vi "Prepare DAQmx Module.vi"(4 "Create Scaling (F)":bool, 6 "On Demand (F)":bool, 8 "error in (no error)":errorcluster, 10 "Group Config (Lookup)":refnum<class "Group Config.lvclass">, 11 "Module in":refnum<class "Module.lvclass">) -> (0 "error out":errorcluster, 1 "Scaling":refnum<class "Scaling.lvclass">, 2 "Group":refnum<class "Group DBL.lvclass">, 3 "Module out":refnum<class "Module.lvclass">, 5 "DAQmx Task":refnum<k21>, 7 "Sampling Config":T1)   [LabVIEW 2023, in "VolatusDAQ.lvlib"]
uses:
  VolatusDAQ.lvlib
  Volatus/Module/Module.lvclass
  lv-vecto/Vecto/Group DBL/Group DBL.lvclass
  VolatusDAQConfig/Sampling Config.ctl
  VolatusData/Scaling/Scaling.lvclass
  Volatus/Event Level.ctl
  Volatus/Module/Module.lvclass/Module.ctl
  VolatusConfig/VolatusConfigElement/VolatusConfigElement.lvclass/VolatusConfigElement.ctl
  Volatus/Module/Config.vi
  VolatusConfig/VolatusConfigElement/Element.vi
  VolatusConfig/Group/Group Config.lvclass
  VolatusConfig/Scaling/Create (Group).vi
  VolatusData/Scaling/Create (Config).vi
  <vilib>/DAQmx/configure/timing.llb/DAQmx Timing (Sample Clock).vi
  VolatusDAQConfig/DAQmxChannel/DAQmxChannel.lvclass
  VolatusConfig/Task/Task Config.lvclass
  VolatusDAQConfig/VolatusDAQConfig.lvlib
  Volatus/Volatus.lvlib
  VolatusConfig/VolatusConfigElement/VolatusConfigElement.lvclass
  VolatusConfig/Channel/Channel Config.lvclass
  C:/dev/volatus/mts-volatus-super/libs/lv-volatus/VolatusConfig/VolatusConfigElement/VolatusConfigElement.lvclass
  C:/dev/volatus/mts-volatus-super/libs/lv-volatus/VolatusConfig/Channel/Channel Config.lvclass
  C:/dev/volatus/mts-volatus-super/libs/lv-vecto/Vecto/Group/Group.lvclass
  C:/dev/volatus/mts-volatus-super/libs/lv-vecto/Vecto/Group DBL/Group DBL.lvclass
  C:/dev/volatus/mts-volatus-super/libs/lv-volatus/VolatusConfig/Group/Group Config.lvclass
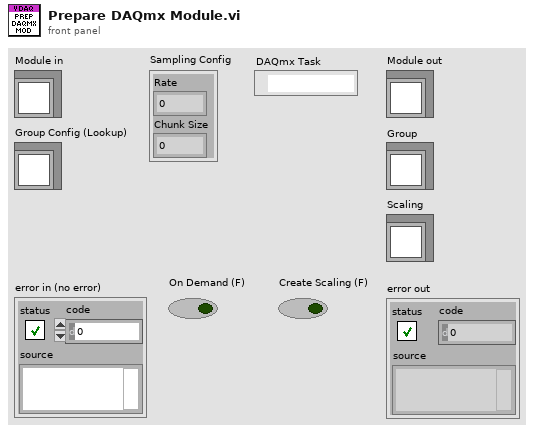
[diagram p1: front panel]
types:
  T1 = typedef "VolatusDAQConfig.lvlib/Sampling Config.ctl" = cluster{"Rate":dbl, "Chunk Size":i32}
  T2 = typedef "Volatus.lvlib/Event Level.ctl" = enum16{"Debug", "Info", "Warning", "Error"}
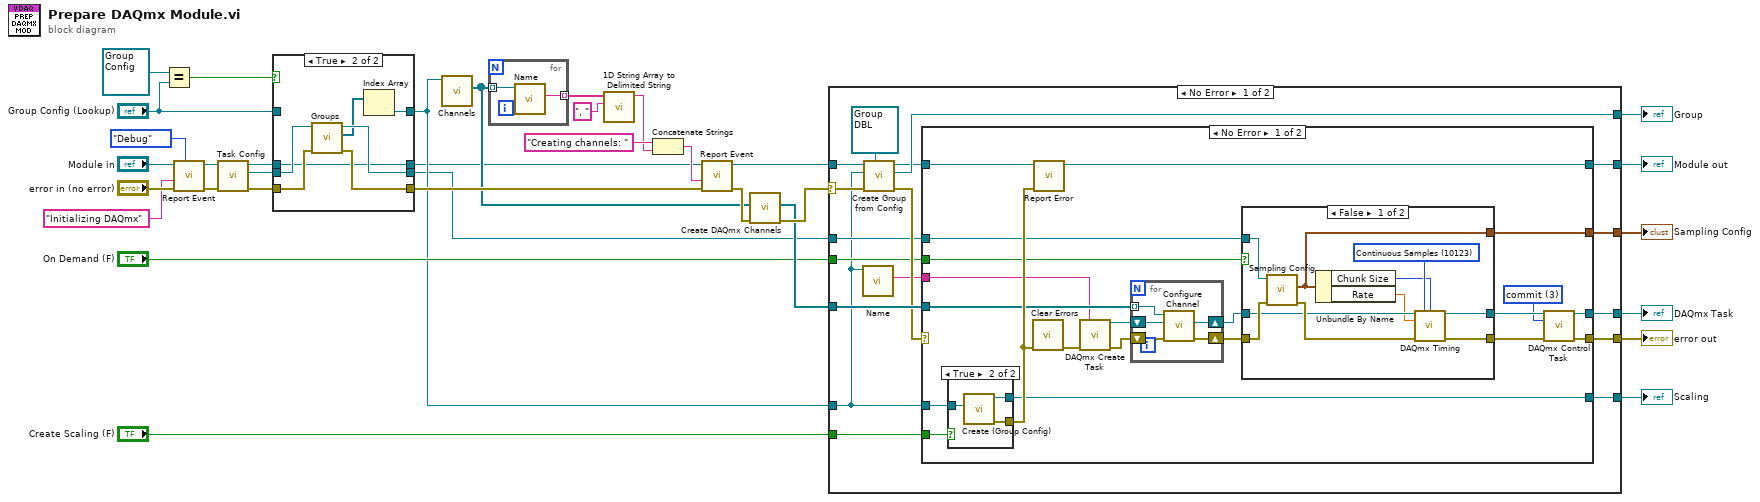
[diagram p0: block diagram]
diagram:
  n1 = Equal?(x=refnum<class "Group Config.lvclass"> refnum, y="Group Config (Lookup)") -> (x = y?=w6:bool)
  n2 = call "Report Event.vi"("Level (Info)"=Event_Level."Debug", "error in (no error)"="error in (no error)", "Message"="Initializing DAQmx", "Module in"="Module in") -> ("error out"=w18:errorcluster, "Module out"=w16:refnum<class "Module.lvclass">)  [unwired: 6 in]
  n3 = call "Task Config.vi"("error in (no error)"=w18, "Module in"=w16) -> ("error out"=w31:errorcluster, "Task Config"=w30:refnum<class "Task Config.lvclass">, "Module out"=w5:refnum<class "Module.lvclass">)  [unwired: 7 in]
  n4 = case shown="True" w6 {
    tunnel: [w36 w45] -> w34
    tunnel: w31 -> [w36 w44]
    tunnel: w30 -> [w35 w43]
    tunnel: [w35 w42] -> w3
    tunnel: [w38 w40] -> w19
    tunnel: "Group Config (Lookup)" -> [w38 _]
    tunnel: w5 -> [w37 w39]
    tunnel: [w37 w39] -> w2
    frame False {
    }
    frame True {
      n5 = call "Groups.vi"("error in (no error)"=w44, "Task in"=w43) -> ("error out"=w45:errorcluster, "Groups"=w41:refnum<class "Group Config.lvclass">[], "Task out"=w42:refnum<class "Task Config.lvclass">)  [unwired: 7 in]
      n6 = Index Array(array=w41) -> (element=w40:refnum<class "Group Config.lvclass">)  [unwired: 1 in]
    }
  }
  n7 = call "Channels.vi"("Group in"=w19) -> ("Channels"=w4:refnum<class "Channel Config.lvclass">[])  [unwired: 8 in, 2 out]
  n8 = for {
    tunnel: w4 -> [w47] mode=indexing
    tunnel: [w46] -> w13 mode=indexing
    n9 = call "Name.vi"("VolatusConfigElement in"=w47) -> ("Name"=w46:string)  [unwired: 8 in, 2 out]
  }
  n10 = call <vilib>:"1D String Array to Delimited String.vi"("delimiter"=", ", "string array"=w13) -> ("delimited string"=w9:string)  [unwired: 9 in]
  n11 = Concatenate Strings("Creating channels: " ("Message"), w9) -> (w8:string)
  n12 = call "Report Event.vi"("error in (no error)"=w34, "Message"=w8, "Module in"=w2) -> ("error out"=w33:errorcluster, "Module out"=w11:refnum<class "Module.lvclass">)  [unwired: 7 in]
  n13 = call "Create DAQmx Channels.vi"("error in (no error)"=w33, "Channels"=w4) -> ("error out"=w32:errorcluster, "DAQmxChannels"=w27:refnum<class "DAQmxChannel.lvclass">[])  [unwired: 8 in]
  n14 = case shown="No Error" w32 {
    selector: w32 -> [w64 w108]
    tunnel: w11 -> [w63 w109]
    tunnel: [w61 _] -> w28
    tunnel: w27 -> [w60 _]
    tunnel: [w59 _] -> w26
    tunnel: [w48 w109] -> w25
    tunnel: [w58 w108] -> w24
    tunnel: [w57 _] -> w23
    tunnel: "Create Scaling (F)" -> [w56 _]
    tunnel: "On Demand (F)" -> [w54 _]
    tunnel: [w53 _] -> w20
    tunnel: w3 -> [w52 _]
    tunnel: w19 -> [w51 _]
    frame No Error {
      n15 = call "Name.vi"("VolatusConfigElement in"=w51) -> ("Name"=w50:string)  [unwired: 8 in, 2 out]
      n16 = call "Create Group from Config.vi"("Group Type (Abstract)"=refnum<class "Group DBL.lvclass"> refnum ("Vecto.lvlib:Group.lvclass"), "error in (no error)"=w64, "Group Config"=w51, "Module in"=w63) -> ("error out"=w55:errorcluster, "Group"=w61:refnum<class "Group DBL.lvclass">, "Module out"=w49:refnum<class "Module.lvclass">)  [unwired: 5 in]
      n17 = case shown="No Error" w55 {
        selector: w55 -> [_ w107]
        tunnel: w60 -> [w79 _]
        tunnel: [w78 _] -> w59
        tunnel: [w77 w107] -> w58
        tunnel: w51 -> [w76 _]
        tunnel: [w75 _] -> w57
        tunnel: w56 -> [w74 _]
        tunnel: w54 -> [w73 _]
        tunnel: [w72 _] -> w53
        tunnel: w52 -> [w71 _]
        tunnel: w50 -> [w69 _]
        tunnel: w49 -> [w67 w106]
        tunnel: [w65 w106] -> w48
        frame No Error {
          w80 = 3 items=["verify"=2, "reserve"=4, "commit"=3, "unreserve"=5, "abort"=6] ("action")
          n18 = case shown="True" w74 {
            tunnel: w76 -> [_ w88]
            tunnel: [_ w87] -> w75
            tunnel: [_ w86] -> w85
            frame False {
            }
            frame True {
              n19 = call "Create (Group Config).vi"("Group Config"=w88) -> ("error out"=w86:errorcluster, "Scaling out"=w87:refnum<class "Scaling.lvclass">)  [unwired: 9 in]
            }
          }
          n20 = call <vilib>:"Clear Errors.vi"("error in (no error)"=w85) -> ("error out"=w66:errorcluster)  [unwired: 5 in, 1 out]
          n21 = call "Report Error.vi"("error in (no error)"=w85, "Module in"=w67) -> ("Module out"=w65:refnum<class "Module.lvclass">)  [unwired: 8 in, 1 out]
          n22 = call <vilib>:"DAQmx Create Task.vi"("new task name"=w69, "error in"=w66) -> ("task out"=w70:refnum<k21>, "error out"=w68:errorcluster)  [unwired: 12 in]
          n23 = for {
            shift-right: [w91] -> w83
            shift-left: w70 -> [w92]
            tunnel: w79 -> [w93] mode=indexing
            shift-right: [w89] -> w84
            shift-left: w68 -> [w90]
            n24 = call-dynamic "Configure Channel.vi"("error in (no error)"=w90, "DAQmx Task In"=w92, "DAQmxChannel in"=w93) -> ("error out"=w89:errorcluster, "DAQmx Task"=w91:refnum<k21>)  [unwired: 7 in]
          }
          n25 = case shown="False" w73 {
            tunnel: w84 -> [w102 w104]
            tunnel: w83 -> [w101 w105]
            tunnel: [w99 w104] -> w82
            tunnel: [w98 w105] -> w81
            tunnel: [w95 _] -> w72
            tunnel: w71 -> [w94 _]
            frame False {
              w100 = 10123 items=["Finite Samples"=10178, "Continuous Samples"=10123, "Hardware Timed Single Point"=12522] ("sample mode")
              n26 = call "Sampling Config.vi"("error in (no error)"=w102, "Task In"=w94) -> ("error out"=w103:errorcluster, "Sampling Config"=w95:T1)  [unwired: 7 in, 1 out]
              n27 = Unbundle By Name(w95) -> ("Chunk Size"=w96:i32, "Rate"=w97:dbl)
              n28 = call-poly <vilib>:"DAQmx Timing.vi"("task/channels in"=w101, "sample mode"=w100, "samples per channel"=w96, "rate"=w97, "error in"=w103) -> ("task out"=w98:refnum<k21>, "error out"=w99:errorcluster)  [unwired: 9 in]
            }
            frame True {
            }
          }
          n29 = call <vilib>:"DAQmx Control Task.vi"("task/channels in"=w81, "action"=w80, "error in"=w82) -> ("task out"=w78:refnum<k21>, "error out"=w77:errorcluster)  [unwired: 11 in]
        }
        frame Error {
        }
      }
    }
    frame Error {
    }
  }
  "Module out" <- w25
  "error out" <- w24
  "Group" <- w28
  "DAQmx Task" <- w26
  "Sampling Config" <- w20
  "Scaling" <- w23
